vi "MissingInProjectCLI.vi"   [LabVIEW 2020, in "Missing in Project Tests.lvlib"]
doc: "Provides a command line interface to the Missing In Project test through G-CLI."
uses:
  Missing in Project Tests.lvlib
  d030f465-a991-474e-afc8-0695029b4070.vi
  <vilib>/Wiresmith Technology/G CLI/CLI Class/CLI.lvclass
types:
  T1 = enum16{"open", "replace", "create", "open or create", "replace or create", "replace or create with confirmation"}
  T2 = enum32{"Invalid", "Standard", "Closed", "Hidden", "Minimized", "Maximized"}
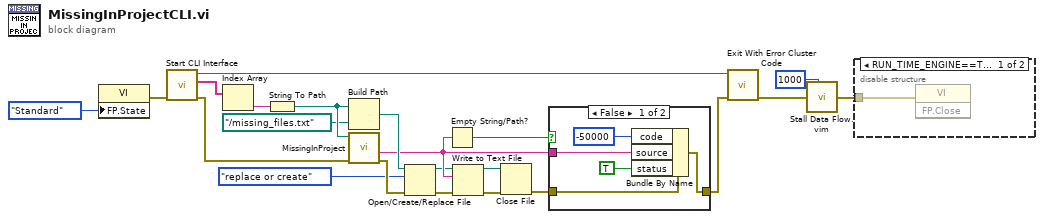
[diagram p0: block diagram]
diagram:
  n1 = property class="VI"("FP.State"=T2."Standard" ("Front Panel Window:State")) -> (error out=w22:errorcluster)  [unwired: 2 in, 1 out]
  n2 = call <vilib>:"Start CLI Interface.vi"("error in (no error)"=w22) -> ("error out"=w21:errorcluster, "Custom Parameters"=w11:string[], "CLI out"=w12:refnum<class "CLI.lvclass">)  [unwired: 7 in, 1 out]
  n3 = Index Array(array=w11) -> (element=w10:string)  [unwired: 1 in]
  n4 = String To Path(string=w10) -> (path=w8:path)
  n5 = Build Path(base path=w8, name or relative path=path "../missing_files.txt") -> (appended path=w6:path)
  n6 = call "MissingInProject.vi"("error in"=w21, "File Path"=w8) -> ("error out"=w18:errorcluster, "Missing Files"=w3:string)  [unwired: 7 in, 1 out]
  n7 = Open/Create/Replace File(file path (use dialog)=w6, error in=w18, operation (0:open)=T1."replace or create") -> (refnum out=w1:refnum<file>, error out=w20:errorcluster)  [unwired: 3 in, 1 out]
  n8 = Empty String/Path?(string/path=w3) -> (empty?=w4:bool)
  n9 = Write to Text File(file (use dialog)=w1, text=w3, error in=w20) -> (refnum out=w9:refnum<file>, error out=w19:errorcluster)  [unwired: 1 in, 1 out]
  n10 = Close File(refnum=w9, error in=w19) -> (error out=w17:errorcluster)  [unwired: 1 out]
  n11 = case shown="False" w4 {
    tunnel: w17 -> [w27 w28]
    tunnel: w3 -> [w24 _]
    tunnel: [w26 w28] -> w16
    frame False {
      n12 = Bundle By Name(cluster=w27, "code"=-50000, "source"=w24, "status"=TRUE) -> (w26:errorcluster)
    }
    frame True {
    }
  }
  n13 = call <vilib>:"Exit With Error Cluster Code.vi"("error in (no error)"=w16, "CLI in"=w12) -> ("error out"=w15:errorcluster)  [unwired: 9 in]
  n14 = call "Stall Data Flow.vim"("value in"=w15, "milliseconds to wait"=u32 1000) -> ("value out"=w14:errorcluster)  [unwired: 1 out]
  n15 = disable-structure shown="RUN_TIME_ENGINE==True" {
    disable-tunnel: w14 -> [w29 _]
    frame condition #0 {
      n16 = invoke class="VI" method="FP.Close"(error in=w29) -> ()  [unwired: 2 in, 3 out]
    }
    frame condition #1 (active) {
    }
  }
